vi "FrequencyShift.vi"(4 "Radio Buttons":T1=enum."Step 1", 5 "AutoCenter":bool, 6 "delta f":dbl, 7 "Deadband":dbl=50.0 format="%#_13g", 8 "ManualShift":dbl, 9 "Shift_":dbl, 10 "NewestPeak":dbl, 11 "Tone.AboveThresh?":bool) -> (1 "TotalShift":dbl)   [LabVIEW 2018]
uses:
  Controls/RadioButtons/FilterEnableRadio.ctl
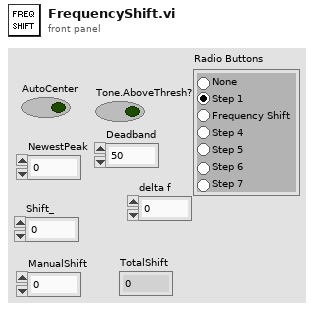
[diagram p1: front panel]
types:
  T1 = typedef "FilterEnableRadio.ctl" = enum32{"None", "Step 1", "Frequency Shift", "Step 4", "Step 5", "Step 6", "Step 7"}
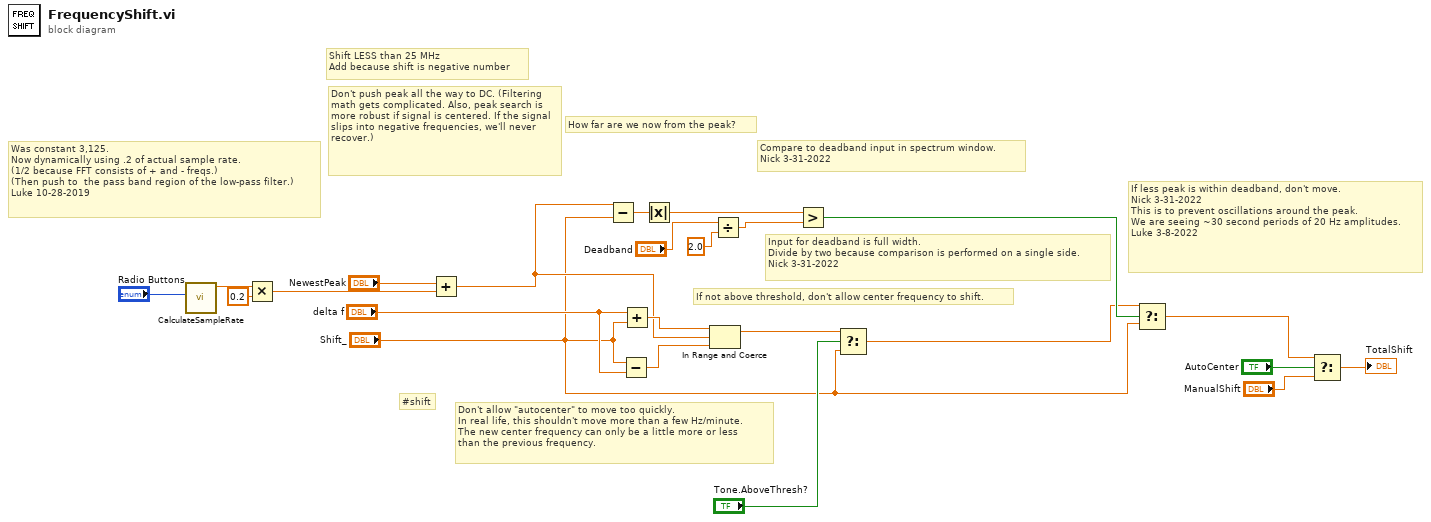
[diagram p0: block diagram]
diagram:
  # "Input for deadband is full width.\nDivide by two because comparison is performed on a single side.\nNick 3-31-2022"
  # "Compare to deadband input in spectrum window.\nNick 3-31-2022"
  # "How far are we now from the peak?"
  # "If less peak is within deadband, don't move.\nNick 3-31-2022\nThis is to prevent oscillations around the peak.\nWe are seeing ~30 second periods of 20 Hz amplitudes.\nLuke 3-8-2022"
  # "If not above threshold, don't allow center frequency to shift."
  # "Was constant 3,125.\nNow dynamically using .2 of actual sample rate.\n(1/2 because FFT consists of + and - freqs.)\n(Then push to  the pass band region of the low-pass filter.)\nLuke 10-28-2019"
  # "#shift"
  # "Don't allow \"autocenter\" to move too quickly. \nIn real life, this shouldn't move more than a few Hz/minute.\nThe new center frequency can only be a little more or less \nthan the previous frequency."
  # "Shift LESS than 25 MHz\nAdd because shift is negative number"
  # "Don't push peak all the way to DC. (Filtering math gets complicated. Also, peak search is more robust if signal is centered. If the signal slips into negative frequencies, we'll never recover.)"
  n1 = call "CalculateSampleRate.vi"("Radio Buttons"="Radio Buttons") -> ("f"=w15:dbl)  [unwired: 10 in]
  n2 = Multiply(x=w15, y=0.2) -> (x*y=w13:dbl)
  n3 = Add(x="NewestPeak", y=w13) -> (x+y=w4:dbl)
  n4 = Subtract(x=w4, y="Shift_") -> (x-y=w10:dbl)
  n5 = Subtract(x="Shift_", y="delta f") -> (x-y=w18:dbl)
  n6 = Add(x="delta f", y="Shift_") -> (x+y=w19:dbl)
  n7 = Absolute Value(x=w10) -> (abs(x)=w9:dbl)
  n8 = In Range and Coerce(upper limit=w19, x=w4, lower limit=w18) -> (coerced(x)=w12:dbl)  [unwired: 1 out]
  n9 = Divide(x="Deadband", y=2.0) -> (x/y=w2:dbl)
  n10 = Greater?(x=w9, y=w2) -> (0:w7:bool)
  n11 = Select(t=w12, s="Tone.AboveThresh?", f="Shift_") -> (s? t:f=w6:dbl)
  n12 = Select(t=w6, s=w7, f="Shift_") -> (s? t:f=w5:dbl)
  n13 = Select(t=w5, s="AutoCenter", f="ManualShift") -> (s? t:f=→"TotalShift":dbl)
